vi "SA5G_getEVM.vi"(8 "error in":errorcluster, 11 "VISA in":refnum<visa-resource-name>) -> (0 "error out":errorcluster, 3 "VISA out":refnum<visa-resource-name>, 4 "get_EVM":T1)   [LabVIEW 2023, in "Keysight.lvlib"]
uses:
  Keysight.lvlib
panel:
  out "subarray":string[](array[string])
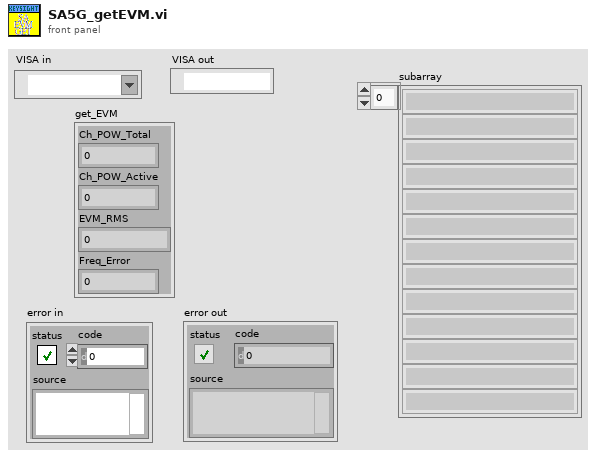
[diagram p1: front panel]
types:
  T1 = cluster{"Ch_POW_Total":dbl, "Ch_POW_Active":dbl, "EVM_RMS":dbl, "Freq_Error":dbl}
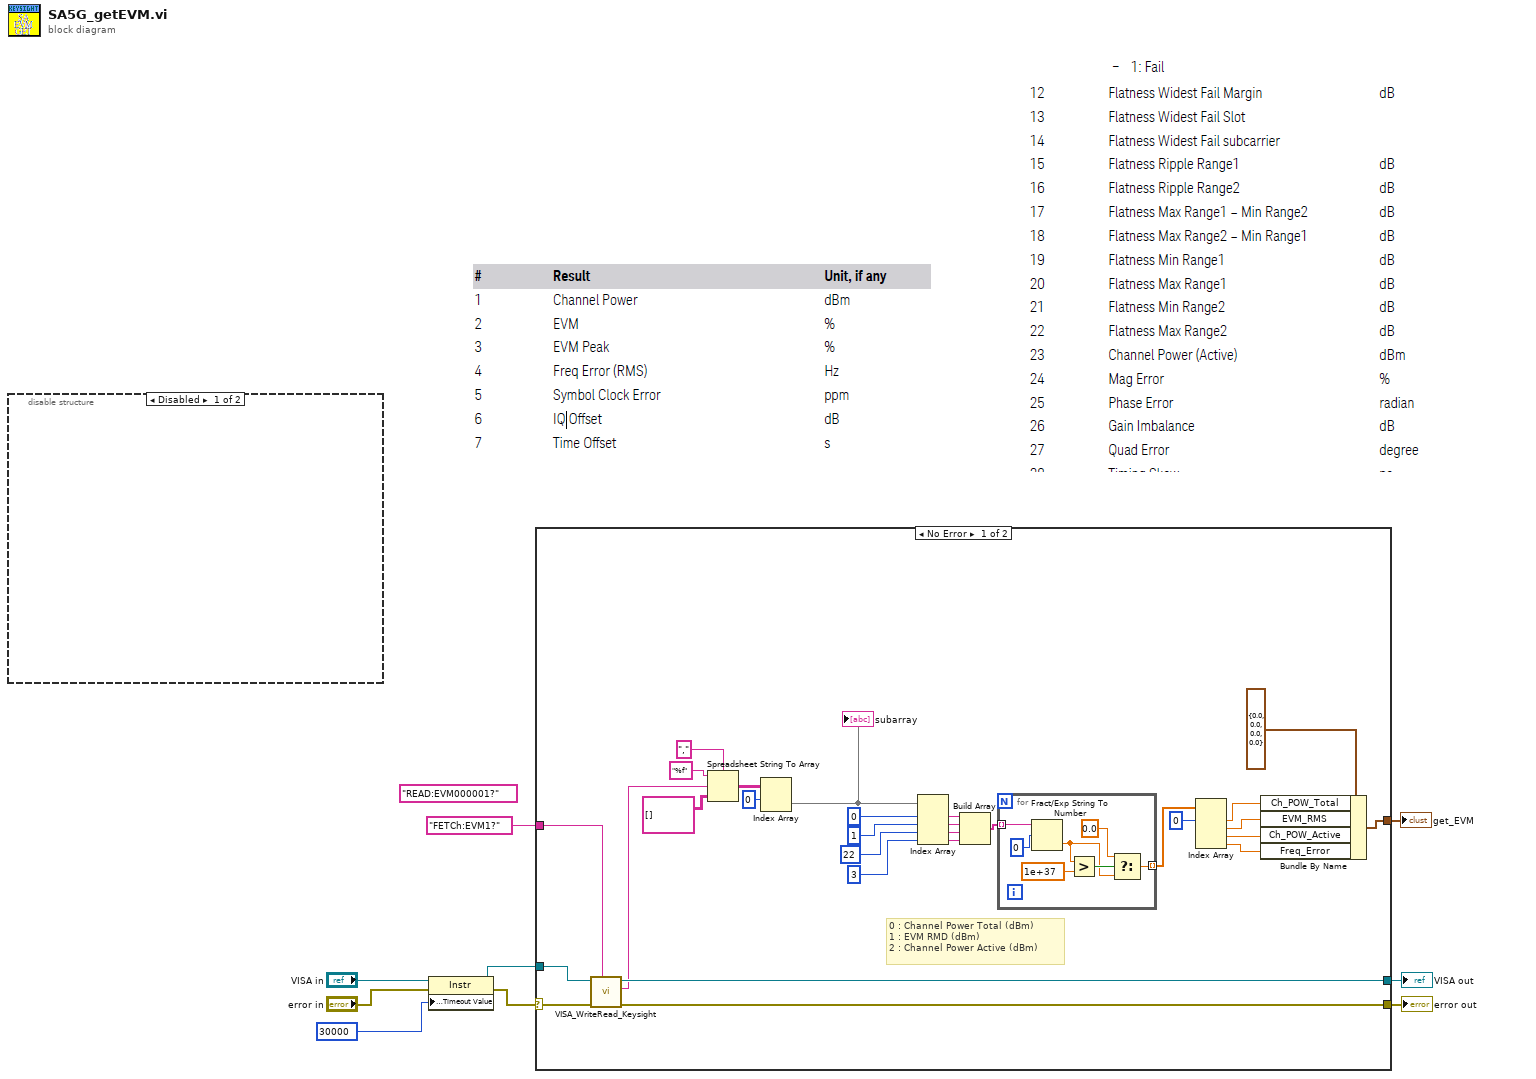
[diagram p0: block diagram]
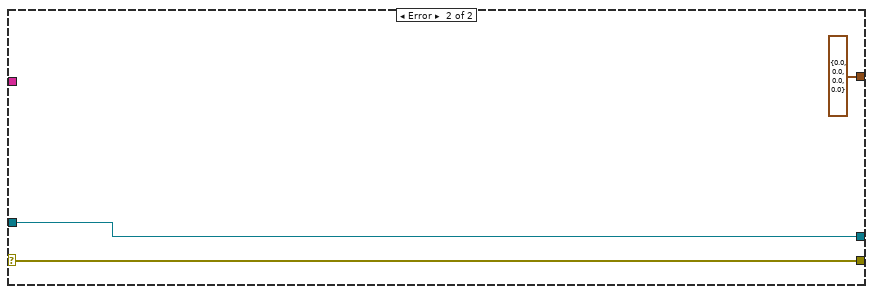
[diagram p3: hidden frame]
diagram:
  (unwired) "READ:EVM000001?" ("write buffer")
  n1 = disable-structure shown="Disabled" {
    frame Disabled {
    }
    frame Enabled {
    }
  }
  n2 = property on="Property Node" class="Instr"(reference="VISA in", error in="error in", "General Settings:Timeout Value"=u32 30000) -> (reference out=w2:refnum<visa-resource-name>, error out=w3:errorcluster)
  n3 = case shown="No Error" w3 {
    selector: w3 -> [w34 w48]
    tunnel: [w38 w48] -> w8
    tunnel: [w37 w47] -> w9
    tunnel: "FETCh:EVM1?" ("write buffer") -> [w36 _]
    tunnel: w2 -> [w35 w47]
    tunnel: [w14 T1 {"Ch_POW_Total"=0.0, "Ch_POW_Active"=0.0, "EVM_RMS"=0.0, "Freq_Error"=0.0} ("get_EVM")] -> w1
    frame No Error {
      # "0 : Channel Power Total (dBm)\n1 : EVM RMD (dBm)\n2 : Channel Power Active (dBm)"
      n4 = call "VISA_WriteRead_Keysight.vi"("VISA_CMD"=w36, "error in"=w34, "VISA in"=w35) -> ("error out"=w38:errorcluster, "Response"=w28:string, "VISA out"=w37:refnum<visa-resource-name>)  [unwired: 6 in]
      n5 = Spreadsheet String To Array(delimiter (Tab)="," ("format string"), format string="%f", spreadsheet string=w28, array type (2D Dbl)=string[][] [] ("Array")) -> (array=w33:string[][])
      n6 = Index Array(array=w33, index (row)=0) -> (element=w27:string[])  [unwired: 1 in]
      "subarray" <- w27
      n7 = Index Array(array=w27, index #1=0 ("index"), index #2=1 ("index"), index #3=22 ("index"), index #4=3 ("index")) -> (element #1=w24:string, element #2=w23:string, element #3=w22:string, element #4=w11:string)
      n8 = Build Array(w24, w23, w22, w11) -> (w21:string[])
      n9 = for {
        tunnel: w21 -> [w40] mode=indexing
        tunnel: [w39] -> w19 mode=indexing
        n10 = Fract/Exp String To Number(string=w40, offset=0) -> (number=w43:dbl)  [unwired: 2 in, 1 out]
        n11 = Greater?(x=w43, y=1e+37 ("number")) -> (0:w44:bool)
        n12 = Select(t=0.0, s=w44, f=w43) -> (s? t:f=w39:dbl)
      }
      n13 = Index Array(array=w19, index #1=0 ("index")) -> (element #1=w17:dbl, element #2=w16:dbl, element #3=w15:dbl, element #4=w10:dbl)  [unwired: 3 in]
      n14 = Bundle By Name(cluster=T1 {"Ch_POW_Total"=0.0, "Ch_POW_Active"=0.0, "EVM_RMS"=0.0, "Freq_Error"=0.0} ("get_EVM"), "Ch_POW_Total"=w17, "EVM_RMS"=w16, "Ch_POW_Active"=w15, "Freq_Error"=w10) -> (w14:T1)
    }
    frame Error {
    }
  }
  "VISA out" <- w9
  "error out" <- w8
  "get_EVM" <- w1
